vi "Get Active Cell Index.vi"(8 "error in (no error)":errorcluster, 11 "DataGridView in":refnum<class "DataGridView.lvclass">) -> (0 "error out":errorcluster, 1 "ColumnIndex":i32, 2 "RowIndex":i32, 3 "DataGridView out":refnum<class "DataGridView.lvclass">)   [LabVIEW 2020, in "DataGrid.lvlib" / "DataGridView.lvclass"]
uses:
  DataGridView.lvclass
  DataGridView.lvclass/DataGridView.ctl
  System.Windows.Forms
  Properties/Read DataGridView.vi
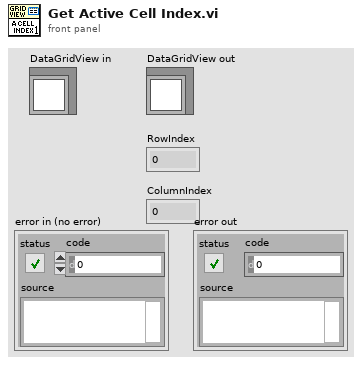
[diagram p1: front panel]
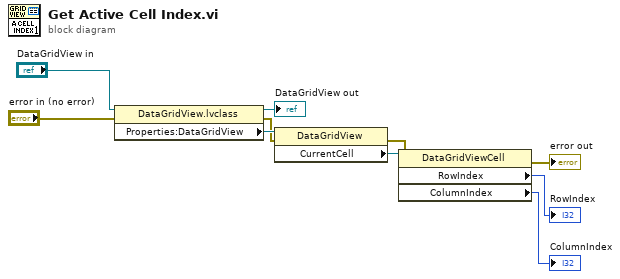
[diagram p0: block diagram]
diagram:
  n1 = property class="DataGridView.lvclass"(reference="DataGridView in", error in="error in (no error)") -> (reference out=→"DataGridView out":refnum<class "DataGridView.lvclass">, error out=w2:errorcluster, "Properties:DataGridView"=w7:refnum<k24>)
  n2 = property class="DataGridView"(reference=w7, error in=w2) -> (error out=w1:errorcluster, "CurrentCell"=w8:refnum<k24>)  [unwired: 1 out]
  n3 = property class="DataGridViewCell"(reference=w8, error in=w1) -> (error out=→"error out":errorcluster, "RowIndex"=→"RowIndex":i32, "ColumnIndex"=→"ColumnIndex":i32)  [unwired: 1 out]
